vi "TrimArray.vi"(10 "曲线点数":i32, 11 "数组输入":dbl[](array[numeric])) -> (3 "数组输出":dbl[](array[numeric]))   [LabVIEW 2018, in "DataDisplay.lvlib"]
uses:
  DataDisplay.lvlib
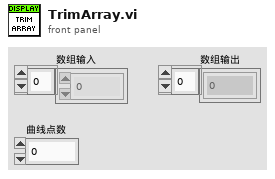
[diagram p1: front panel]
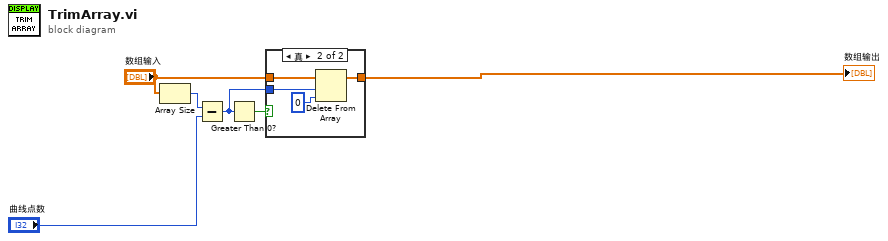
[diagram p0: block diagram]
diagram:
  n1 = Array Size(array="数组输入") -> (size(s)=w3:i32)
  n2 = Subtract(x=w3, y="曲线点数") -> (x-y=w5:i32)
  n3 = Greater Than 0?(x=w5) -> (x > 0?=w4:bool)
  n4 = case shown="真" w4 {
    tunnel: "数组输入" -> [w7 w11]
    tunnel: w5 -> [_ w9]
    tunnel: [w7 w8] -> w1
    frame False {
    }
    frame True {
      n5 = Delete From Array(array=w11, length=w9, index=0 ("索引")) -> (array with subset deleted=w8:dbl[])  [unwired: 1 out]
    }
  }
  "数组输出" <- w1
